vi "Get Azimut.vi"(9 "Transformation Matrix":T1, 10 "Final":cluster{"X":dbl, "Y":dbl}, 11 "Initial":cluster{"X":dbl, "Y":dbl}) -> (2 "Angle [deg]":dbl, 3 "Angle [rad]":dbl)   [LabVIEW 2012, in "Targeting Unit.lvlib"]
uses:
  <vilib>/Analysis/Matrix/Datatypes/RealMatrix.ctl
  Targeting Unit.lvlib
  <vilib>/Analysis/Matrix/NI_Matrix.lvlib
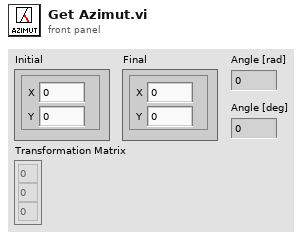
[diagram p1: front panel]
types:
  T1 = typedef "NI_Matrix.lvlib/RealMatrix.ctl" = dbl[][]
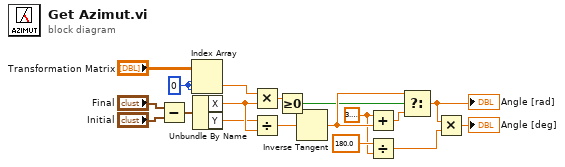
[diagram p0: block diagram]
diagram:
  w16 = 0 ("index (row)")
  w4 = 3.141592653589793
  n1 = Subtract(x="Final", y="Initial") -> (x-y=w12:cluster{"X":dbl, "Y":dbl})
  n2 = Index Array(array="Transformation Matrix", index (row)=w16, index (col)=w16) -> (element=w18:dbl)
  n3 = Unbundle By Name(w12) -> ("X"=w15:dbl, "Y"=w13:dbl)
  n4 = Multiply(x=w18, y=w15) -> (x*y=w14:dbl)
  n5 = Divide(x=w13, y=w15) -> (x/y=w10:dbl)
  n6 = Greater Or Equal To 0?(x=w14) -> (x >= 0?=w8:bool)
  n7 = Inverse Tangent(1:w10) -> (0:w9:dbl)
  n8 = Add(x=w4, y=w9) -> (x+y=w7:dbl)
  n9 = Divide(x=180.0, y=w4) -> (x/y=w1:dbl)
  n10 = Select(t=w9, s=w8, f=w7) -> (s? t:f=w2:dbl)
  "Angle [rad]" <- w2
  n11 = Multiply(x=w2, y=w1) -> (x*y=→"Angle [deg]":dbl)
